vi "p1.vi"() -> ()   [LabVIEW 2021, in "d8.lvlib"]
uses:
  d8.lvlib
  AOC/AOC.lvlib
panel:
  in  "Example":string="30373\n25512\n65332\n33549\n35390"
  in  "Example":bool
  out "Answer":i64=1719
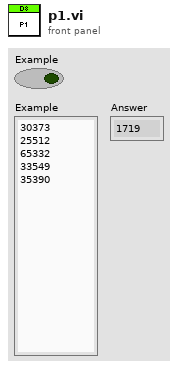
[diagram p1: front panel]
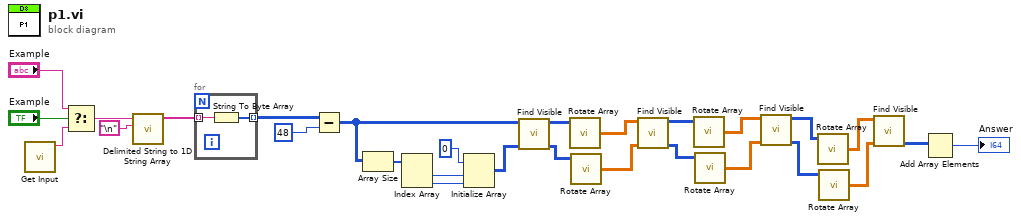
[diagram p0: block diagram]
diagram:
  n1 = call "Get Input.vi"() -> ("Input"=w28:string)  [unwired: 11 in]
  n2 = Select(t="Example", s="Example", f=w28) -> (s? t:f=w27:string)
  n3 = call <vilib>:"Delimited String to 1D String Array.vi"("delimiter"="\n", "delimited string"=w27) -> ("string array"=w23:string[])  [unwired: 9 in]
  n4 = for {
    tunnel: w23 -> [w30] mode=indexing
    tunnel: [w29] -> w22 mode=indexing
    n5 = String To Byte Array(string=w30) -> (unsigned byte array=w29:u8[])
  }
  n6 = Subtract(x=w22, y=u8 48) -> (x-y=w17:u8[][])
  n7 = Array Size(array=w17) -> (size(s)=w20:i32[])
  n8 = Index Array(array=w20) -> (element #1=w19:i32, element #2=w18:i32)  [unwired: 2 in]
  n9 = Initialize Array(i16 0 ("Visible in"), w19, w18) -> (w14:i16[][])
  n10 = call "Find Visible.vi"("Visible in"=w14, "Height in"=w17) -> ("Visible in"=w13:i16[][], "Height out"=w16:u8[][])  [unwired: 8 in]
  n11 = call "Rotate Array.vi"("Array"=w16) -> ("Rotated 2D Array"=w12:dbl[][])  [unwired: 2 in]
  n12 = call "Rotate Array.vi"("Array"=w13) -> ("Rotated 2D Array"=w11:dbl[][])  [unwired: 2 in]
  n13 = call "Find Visible.vi"("Visible in"=w11, "Height in"=w12) -> ("Visible in"=w9:i16[][], "Height out"=w10:u8[][])  [unwired: 8 in]
  n14 = call "Rotate Array.vi"("Array"=w10) -> ("Rotated 2D Array"=w8:dbl[][])  [unwired: 2 in]
  n15 = call "Rotate Array.vi"("Array"=w9) -> ("Rotated 2D Array"=w7:dbl[][])  [unwired: 2 in]
  n16 = call "Find Visible.vi"("Visible in"=w7, "Height in"=w8) -> ("Visible in"=w5:i16[][], "Height out"=w6:u8[][])  [unwired: 8 in]
  n17 = call "Rotate Array.vi"("Array"=w6) -> ("Rotated 2D Array"=w4:dbl[][])  [unwired: 2 in]
  n18 = call "Rotate Array.vi"("Array"=w5) -> ("Rotated 2D Array"=w3:dbl[][])  [unwired: 2 in]
  n19 = call "Find Visible.vi"("Visible in"=w3, "Height in"=w4) -> ("Visible in"=w2:i16[][])  [unwired: 8 in, 1 out]
  n20 = Add Array Elements(numeric array=w2) -> (sum=→"Answer":i16)
